vi "vision.vi"() -> ()   [LabVIEW 2018]
panel:
  out "Image":T1(plugin-control)
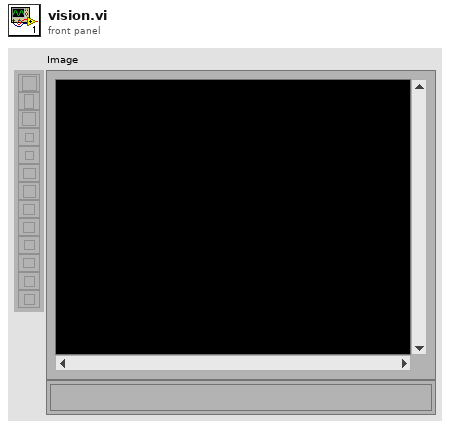
[diagram p1: front panel]
types:
  T1 = typedef "IMAQ Image.ctl" = refnum<image>
  T2 = typedef "VBAIInterface.ctl" = refnum<k21>
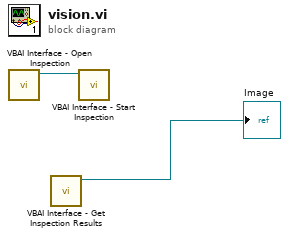
[diagram p0: block diagram]
diagram:
  n1 = call <vilib>:"VBAI Interface - Open Inspection.vi"() -> ("Session Out"=w3:T2)  [unwired: 10 in, 1 out]
  n2 = call <vilib>:"VBAI Interface - Get Inspection Results.vi"() -> ("Session Out"=→"Image":T2)  [unwired: 5 in, 6 out]
  n3 = call <vilib>:"VBAI Interface - Start Inspection.vi"("Session In"=w3) -> ("Session Out"=w1:T2)  [unwired: 9 in, 1 out]
